vi "File.CSV to String Array.vi"(7 "Remove Quotes":bool=TRUE, 8 "error in":errorcluster, 10 "Separate Header Row":bool=TRUE, 11 "File":path=path "C:/Users/eddiek/Documents/01_MTE/Circle Test/Results/ATS_TL/Circle Test Summary Data, 10-06-2017/AB736001B5_CT02_CS01.csv") -> (0 "error out":errorcluster, 1 "Top Row (Header)":string[](array[string]), 2 "2D Array":string[][](array[string]), 3 "Dup File":path)   [LabVIEW 2018]
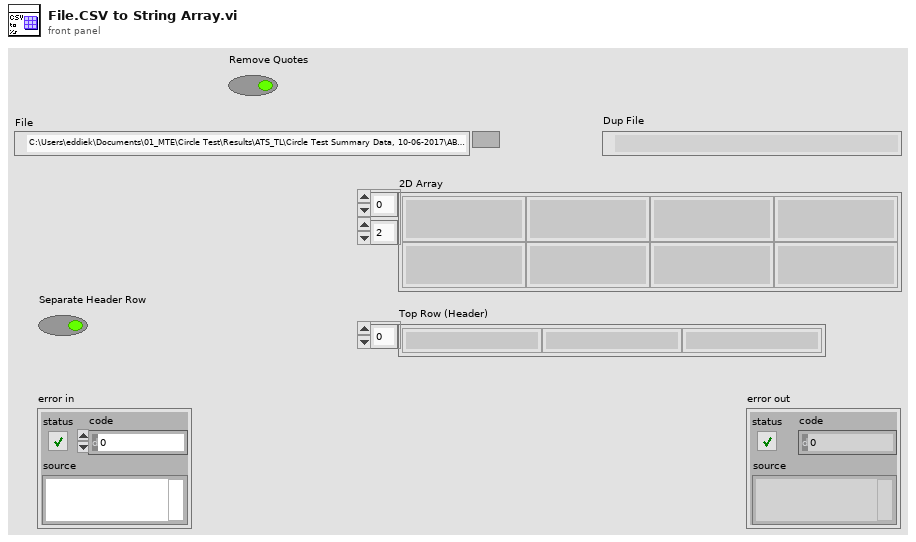
[diagram p1: front panel]
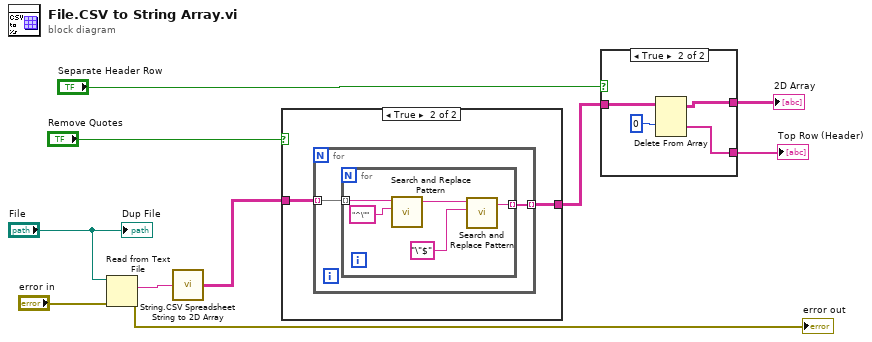
[diagram p0: block diagram]
diagram:
  n1 = Read from Text File(file (use dialog)="File", error in="error in") -> (text=w5:string, error out=→"error out":errorcluster)  [unwired: 2 in, 2 out]
  n2 = call "String.CSV Spreadsheet String to 2D Array.vi"("CSV Data"=w5) -> ("2D Data"=w3:string[][])
  n3 = case shown="True" "Remove Quotes" {
    tunnel: w3 -> [w11 w13]
    tunnel: [w11 w12] -> w2
    frame False {
    }
    frame True {
      n4 = for {
        tunnel: w13 -> [w15] mode=indexing
        tunnel: [w14] -> w12 mode=indexing
        n5 = for {
          tunnel: w15 -> [w20] mode=indexing
          tunnel: [w16] -> w14 mode=indexing
          n6 = call <vilib>:"Search and Replace Pattern.vi"("string"=w20, "regular expression (\"\")"="^\"" ("regular expression (\"\")")) -> ("result string"=w17:string)  [unwired: 3 in, 1 out]
          n7 = call <vilib>:"Search and Replace Pattern.vi"("string"=w17, "regular expression (\"\")"="\"$" ("regular expression (\"\")")) -> ("result string"=w16:string)  [unwired: 3 in, 1 out]
        }
      }
    }
  }
  n8 = case shown="True" "Separate Header Row" {
    tunnel: w2 -> [w21 w25]
    tunnel: [w21 w24] -> w10
    tunnel: [_ w23] -> w9
    frame False {
    }
    frame True {
      n9 = Delete From Array(array=w25, index (row)=0 ("length")) -> (deleted portion=w23:string[], array with subset deleted=w24:string[][])  [unwired: 2 in]
    }
  }
  "2D Array" <- w10
  "Top Row (Header)" <- w9
  "Dup File" <- "File"
